vi "list and create PG table.vi"(6 "columns type (real)":string="real", 8 "error in":errorcluster, 9 "columns":string[](array[string]), 10 "table name":string, 11 "conn":u64) -> (0 "error out":errorcluster, 3 "conn_out":u64)   [LabVIEW 2019, in "PostgreSQL.lvlib"]
uses:
  PostgreSQL.lvlib
  PostgreSQL2LabVIEW/libpqlv64/src/PQresultErrorMessage.vi
  PostgreSQL2LabVIEW/libpqUtility64/src/PQclear.vi
  PostgreSQL2LabVIEW/libpqlv64/src/PQsendQuery.vi
  PostgreSQL2LabVIEW/libpqlv64/src/PQgetResult.vi
  PostgreSQL2LabVIEW/libpqlv64/src/PQresultStatus.vi
  PostgreSQL2LabVIEW/libpqUtility64/src/PQgetColumn.vi
  PostgreSQL2LabVIEW/libpqlv64/src/PQclear.vi
  PostgreSQL2LabVIEW/libpqUtility64/src/PQfetchTables.vi
  PostgreSQL2LabVIEW/libpqlv64/src/PQgetvalue.vi
  PostgreSQL2LabVIEW/libpqlv64/src/PQntuples.vi
  PostgreSQL2LabVIEW/libpqUtility64/libpqutility64.lvlib
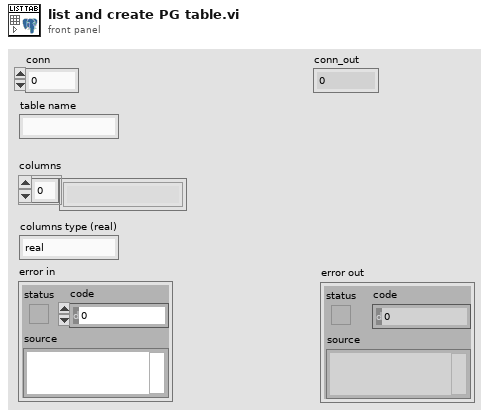
[diagram p1: front panel]
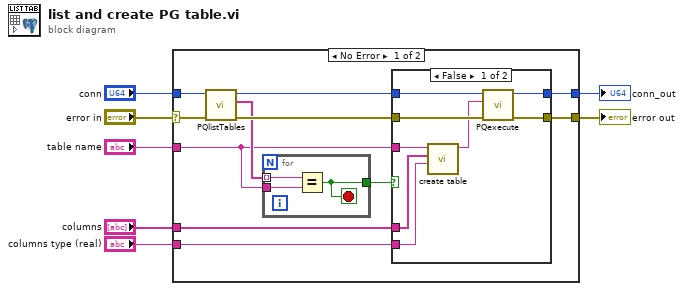
[diagram p0: block diagram]
diagram:
  n1 = case shown="No Error" "error in" {
    selector: "error in" -> [w15 w33]
    tunnel: "conn" -> [w12 w32]
    tunnel: [w18 w32] -> w5
    tunnel: "columns" -> [w9 _]
    tunnel: [w17 w33] -> w4
    tunnel: "table name" -> [w10 _]
    tunnel: "columns type (real)" -> [w8 _]
    frame No Error {
      n2 = call "PQlistTables.vi"("error in"=w15, "conn"=w12) -> ("error out"=w14:errorcluster, "Data"=w11:string[], "conn_out"=w13:u64)  [unwired: 7 in]
      n3 = for {
        tunnel: w10 -> [w20]
        tunnel: w11 -> [w21] mode=indexing
        tunnel: [w19] -> w16
        stop <- w19 stop-if-true
        n4 = Equal?(x=w21, y=w20) -> (x = y?=w19:bool)
      }
      n5 = case shown="False" w16 {
        tunnel: w13 -> [w27 w31]
        tunnel: [w24 w31] -> w18
        tunnel: w14 -> [w26 w30]
        tunnel: [w23 w30] -> w17
        tunnel: w9 -> [w28 _]
        tunnel: w10 -> [w29 _]
        tunnel: w8 -> [w22 _]
        frame False {
          n6 = call "create table.vi"("columns type (real)"=w22, "columns"=w28, "table name"=w29) -> ("create table parameters"=w25:string)  [unwired: 8 in]
          n7 = call "PQexecute.vi"("error in"=w26, "SQL querry"=w25, "conn"=w27) -> ("error out"=w23:errorcluster, "conn_out"=w24:u64)  [unwired: 7 in]
        }
        frame True {
        }
      }
    }
    frame Error {
    }
  }
  "conn_out" <- w5
  "error out" <- w4
